vi "TailInsertionBenchmark_NativeArray.vi"() -> ()   [LabVIEW 2013]
panel:
  out "Array":string[](array[string])
  in  "Number of Elements":i32
  out "Native Array":u32
  # "Tail Insertion - Native Array"
  # "100,000 to 500,000 elements is sufficient to see the difference in time for each of the implementations."
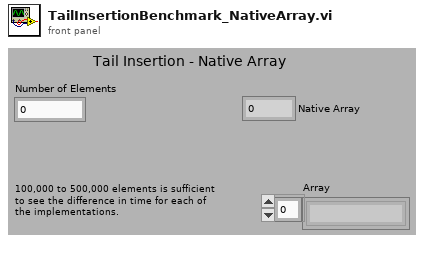
[diagram p1: front panel]
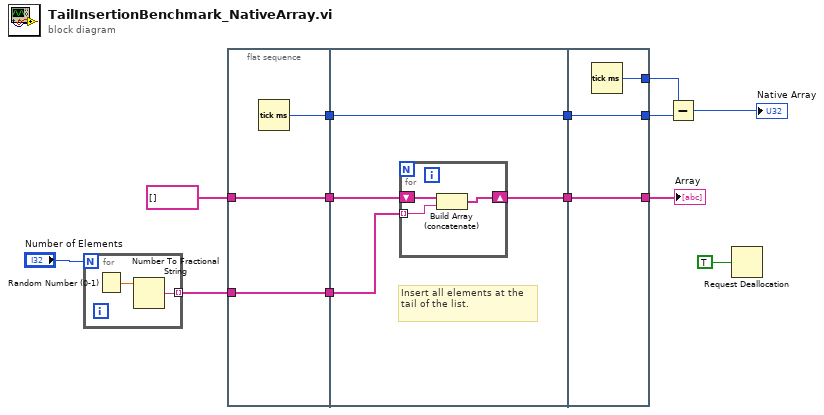
[diagram p0: block diagram]
diagram:
  n1 = for {
    N: "Number of Elements" -> [_]
    tunnel: [w14] -> w12 mode=indexing
    n2 = Random Number (0-1)() -> (number: 0 to 1=w15:dbl)
    n3 = Number To Fractional String(number=w15) -> (F-format string=w14:string)  [unwired: 3 in]
  }
  n4 = flat-sequence {
    tunnel: w12 -> [w18]
    tunnel: [w18] -> w11
    tunnel: [w17] -> w10
    tunnel: [w16] -> w9
    tunnel: string[] [] -> [w16]
    tunnel: w11 -> [w22]
    tunnel: w10 -> [w19]
    tunnel: w9 -> [w21]
    tunnel: [w20] -> w8
    tunnel: [w19] -> w7
    tunnel: [w28] -> w1
    tunnel: w8 -> [w28]
    tunnel: w7 -> [w26]
    tunnel: [w27] -> w6
    tunnel: [w26] -> w5
    frame #0 {
      n5 = Tick Count (ms)() -> (millisecond timer value=w17:u32)
    }
    frame #1 {
      # "Insert all elements at the tail of the list."
      n6 = for {
        shift-right: [w24] -> w20
        shift-left: w21 -> [w25]
        tunnel: w22 -> [w23] mode=indexing
        n7 = Build Array (concatenate)(w25, w23) -> (w24:string[])
      }
    }
    frame #2 {
      n8 = Tick Count (ms)() -> (millisecond timer value=w27:u32)
    }
  }
  n9 = Subtract(x=w6, y=w5) -> (x-y=→"Native Array":u32)
  n10 = Request Deallocation(TRUE ("flag")) -> ()
  "Array" <- w1
